vi "Assign Y Coordinate and Width.vi"(5 "Width Padding":i32, 7 "[user-specified font]":T5, 8 "Leaf Width":i32=16, 9 "Row Gap":i32=40, 10 "Max Height per Row":dbl[](array[numeric]), 11 "Tree with Heights in":T1) -> (3 "Decision Tree Out":T1)   [LabVIEW 2025]
uses:
  Types/Decision Tree.ctl
  Types/Sequencing Tree Node.ctl
  Types/Single Cmd Info.ctl
  <vilib>/picture/picture.llb/imagedata.ctl
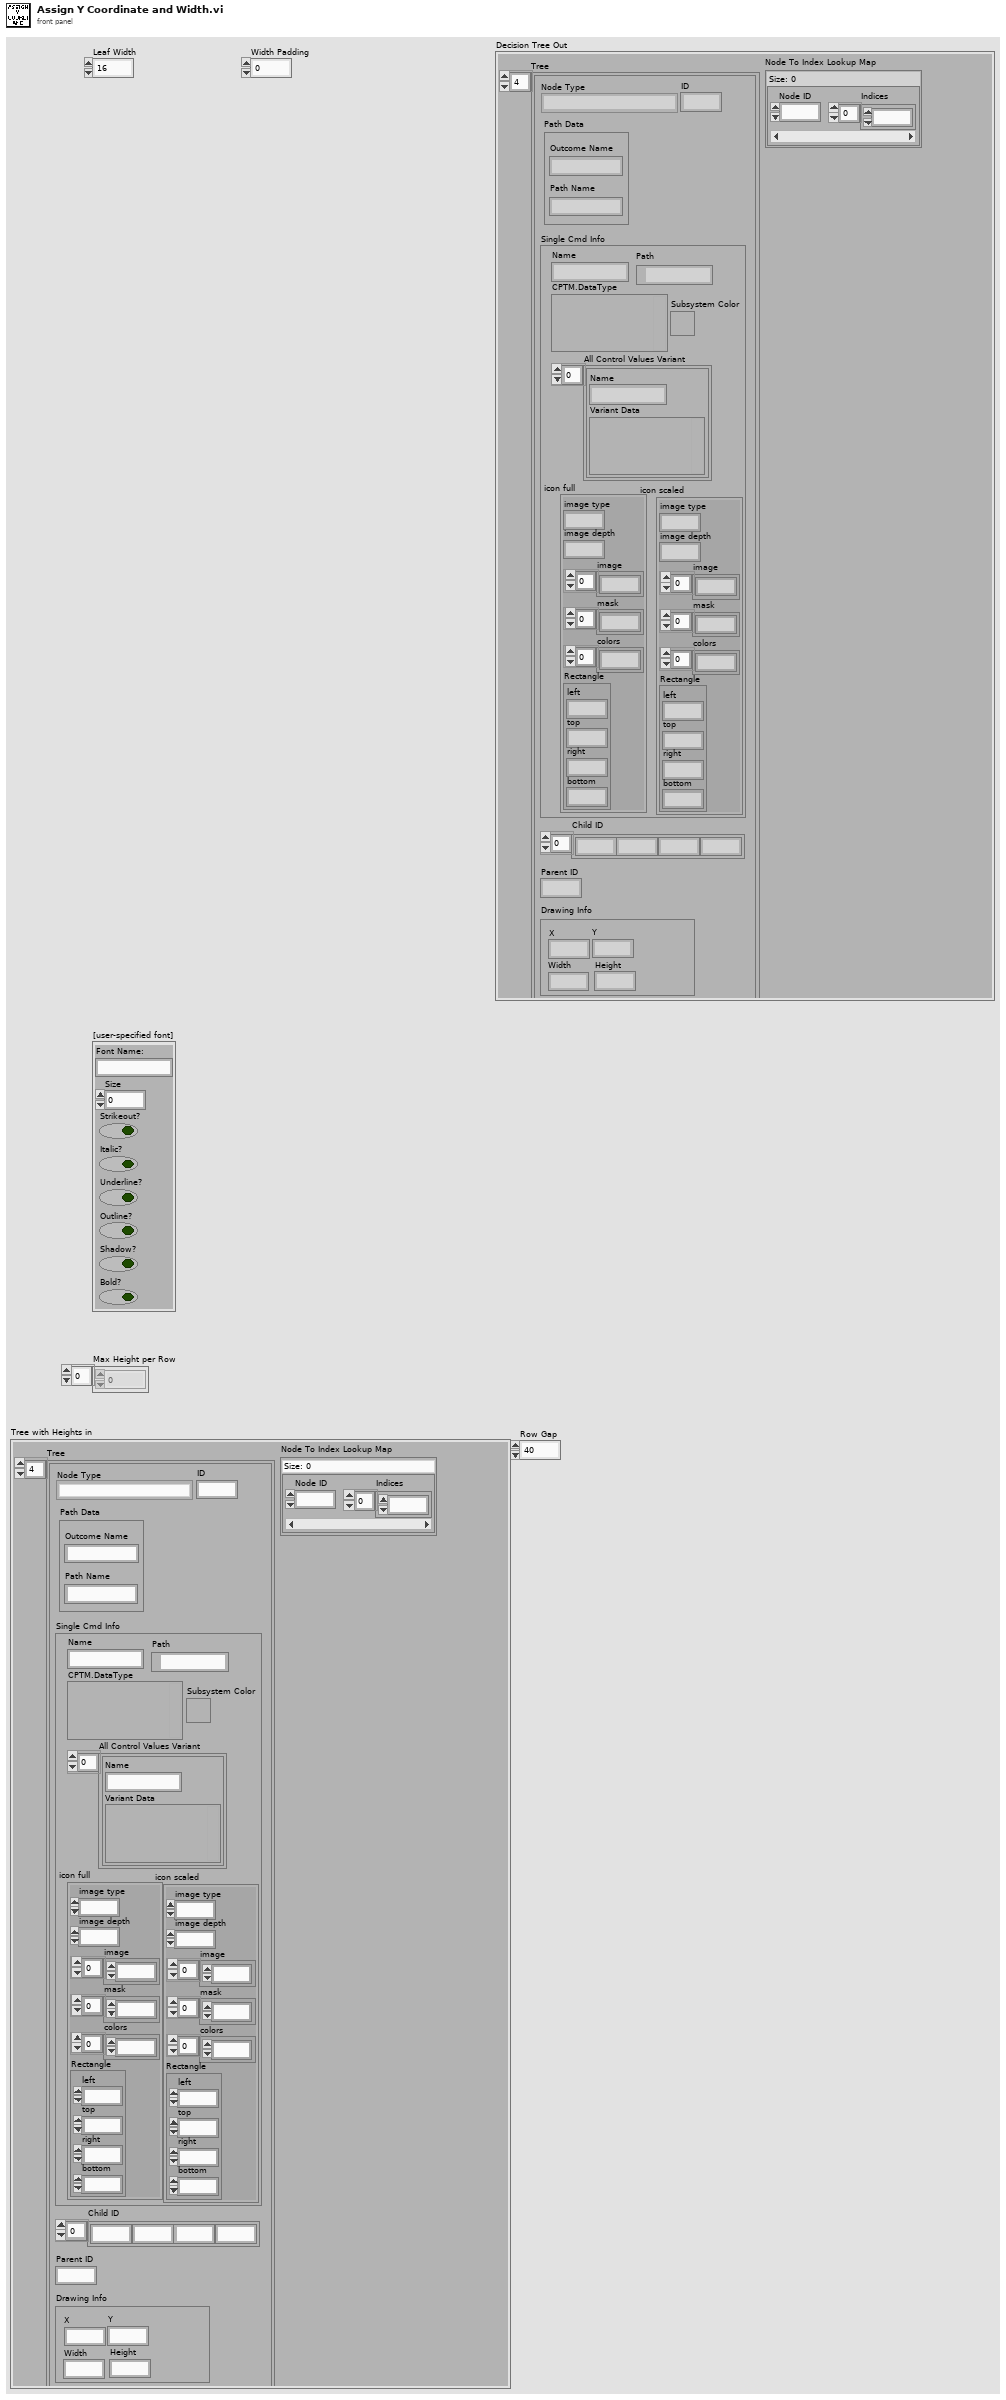
[diagram p1: front panel]
types:
  T1 = typedef "Decision Tree.ctl" = cluster{"Tree":T2[], "Node To Index Lookup Map":map{i16, i16[]}}
  T2 = typedef "Sequencing Tree Node.ctl" = cluster{"Node Type":enum16{"Path", "Command", "Leaf"}, "ID":i16, "Path Data":cluster{"Path Name":string, "Outcome Name":string}, "Single Cmd Info":T3, "Child ID":i32[], "Parent ID":i32, "Drawing Info":cluster{"X":i32, "Y":i32, "Width":i32, "Height":i32}}
  T3 = typedef "Single Cmd Info.ctl" = cluster{"Name":string, "CPTM.DataType":variant, "All Control Values Variant":cluster{"Name":string, "Variant Data":variant}[], "icon full":T4, "icon scaled":T4, "Path":path, "Subsystem Color":u32}
  T4 = typedef "imagedata.ctl" = cluster{"image type":i32, "image depth":i32, "image":u8[], "mask":u8[], "colors":u32[], "Rectangle":cluster{"left":i16, "top":i16, "right":i16, "bottom":i16}}
  T5 = cluster{"Font Name:":string, "Size":i16, "Strikeout?":bool, "Italic?":bool, "Underline?":bool, "Outline?":bool, "Shadow?":bool, "Bold?":bool}
  T6 = enum16{"User-specified Font", "Application Font", "System Font", "Dialog Font"}
  T7 = cluster{"Path Name":string, "Outcome Name":string}
  T8 = cluster{"X":i32, "Y":i32, "Width":i32, "Height":i32}
  T9 = cluster{"left":i16, "top":i16, "right":i16, "bottom":i16}
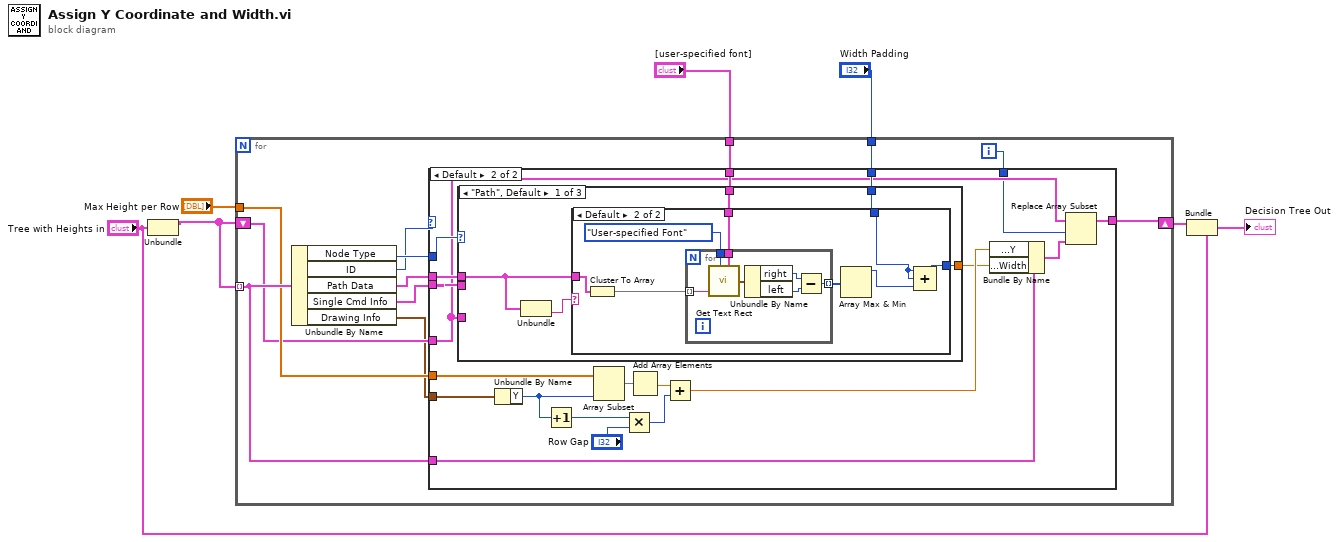
[diagram p0: block diagram]
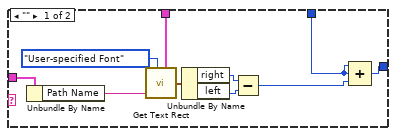
[diagram p3: hidden frame]
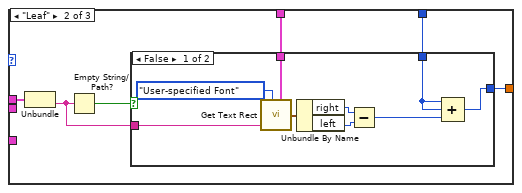
[diagram p4: hidden frame]
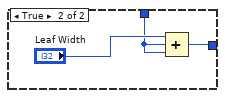
[diagram p5: hidden frame]
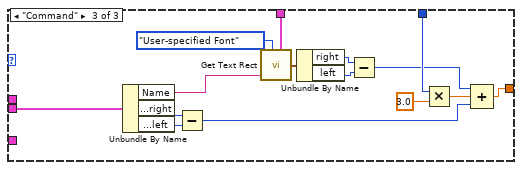
[diagram p6: hidden frame]
diagram:
  n1 = Unbundle("Tree with Heights in") -> ("Tree"=w4:T2[])  [unwired: 1 out]
  n2 = for {
    tunnel: w4 -> [w18] mode=indexing
    tunnel: "Max Height per Row" -> [w17]
    tunnel: "Width Padding" -> [w15]
    tunnel: "[user-specified font]" -> [w14]
    shift-right: [w11] -> w2
    shift-left: w4 -> [w12]
    i -> [w8]
    n3 = Unbundle By Name(w18) -> ("Node Type"=w19:enum16{"Path", "Command", "Leaf"}, "ID"=w10:i16, "Path Data"=w13:T7, "Single Cmd Info"=w16:T3, "Drawing Info"=w9:T8)
    n4 = case shown="Default" w10 {
      tunnel: w19 -> [_ w40]
      tunnel: w18 -> [_ w39]
      tunnel: w9 -> [_ w38]
      tunnel: w17 -> [_ w37]
      tunnel: w16 -> [_ w31]
      tunnel: w15 -> [_ w30]
      tunnel: w14 -> [_ w29]
      tunnel: w13 -> [_ w27]
      tunnel: w12 -> [w20 w26]
      tunnel: [w20 w24] -> w11
      tunnel: w8 -> [_ w21]
      frame -1 {
      }
      frame Default {
        n5 = case shown="\"Path\", Default" w40 {
          tunnel: w31 -> [_ _ w103]
          tunnel: w30 -> [w45 w72 w99]
          tunnel: w29 -> [w44 w73 w98]
          tunnel: [w43 w74 w92] -> w28
          tunnel: w26 -> [_ _ _]
          tunnel: w27 -> [w42 w76 _]
          frame "Path", Default {
            n6 = Unbundle(w42) -> ("Outcome Name"=w41:string)  [unwired: 1 out]
            n7 = case shown="Default" w41 {
              tunnel: w45 -> [w46 w56]
              tunnel: w44 -> [w51 w62]
              tunnel: w42 -> [w50 w61]
              tunnel: [w48 w58] -> w43
              frame "" {
                n8 = Unbundle By Name(w50) -> ("Path Name"=w49:string)
                n9 = call <vilib>:"Get Text Rect.vi"("desired font(Application)"=T6."User-specified Font", "text"=w49, "[user-specified font]"=w51) -> ("rect"=w54:T9)  [unwired: 6 in]
                n10 = Unbundle By Name(w54) -> ("right"=w53:i16, "left"=w52:i16)
                n11 = Subtract(x=w53, y=w52) -> (x-y=w47:i16)
                n12 = Compound Arithmetic op=ADD(w46, w46, w47) -> (w48:i32)
              }
              frame Default {
                n13 = Cluster To Array(cluster=w61) -> (array=w60:string[])
                n14 = for {
                  tunnel: T6."User-specified Font" ("desired font(Application)") -> [w70]
                  tunnel: [w66] -> w59 mode=indexing
                  tunnel: w62 -> [w65]
                  tunnel: w60 -> [w64] mode=indexing
                  n15 = call <vilib>:"Get Text Rect.vi"("desired font(Application)"=w70, "text"=w64, "[user-specified font]"=w65) -> ("rect"=w69:T9)  [unwired: 6 in]
                  n16 = Unbundle By Name(w69) -> ("right"=w68:i16, "left"=w67:i16)
                  n17 = Subtract(x=w68, y=w67) -> (x-y=w66:i16)
                }
                n18 = Array Max & Min(array=w59) -> (max value=w57:i16)  [unwired: 3 out]
                n19 = Compound Arithmetic op=ADD(w56, w56, w57) -> (w58:i32)
              }
            }
          }
          frame "Leaf" {
            n20 = Unbundle(w76) -> ("Outcome Name"=w71:string)  [unwired: 1 out]
            n21 = Empty String/Path?(string/path=w71) -> (empty?=w75:bool)
            n22 = case shown="False" w75 {
              tunnel: [w79 w87] -> w74
              tunnel: w73 -> [w81 _]
              tunnel: w72 -> [w78 w86]
              tunnel: w71 -> [w77 _]
              frame False {
                n23 = call <vilib>:"Get Text Rect.vi"("desired font(Application)"=T6."User-specified Font", "text"=w77, "[user-specified font]"=w81) -> ("rect"=w84:T9)  [unwired: 6 in]
                n24 = Unbundle By Name(w84) -> ("right"=w83:i16, "left"=w82:i16)
                n25 = Subtract(x=w83, y=w82) -> (x-y=w80:i16)
                n26 = Compound Arithmetic op=ADD(w78, w78, w80) -> (w79:i32)
              }
              frame True {
                n27 = Compound Arithmetic op=ADD("Leaf Width", w86, w86) -> (w87:i32)
              }
            }
          }
          frame "Command" {
            n28 = Unbundle By Name(w103) -> ("Name"=w96:string, "icon scaled.Rectangle.right"=w102:i16, "icon scaled.Rectangle.left"=w101:i16)
            n29 = Subtract(x=w102, y=w101) -> (x-y=w91:i16)
            n30 = call <vilib>:"Get Text Rect.vi"("desired font(Application)"=T6."User-specified Font", "text"=w96, "[user-specified font]"=w98) -> ("rect"=w95:T9)  [unwired: 6 in]
            n31 = Unbundle By Name(w95) -> ("right"=w94:i16, "left"=w93:i16)
            n32 = Subtract(x=w94, y=w93) -> (x-y=w89:i16)
            n33 = Multiply(x=w99, y=3.0) -> (x*y=w90:dbl)
            n34 = Compound Arithmetic op=ADD(w89, w90, w91) -> (w92:dbl)
          }
        }
        n35 = Unbundle By Name(w38) -> ("Y"=w22:i32)
        n36 = Increment(x=w22) -> (x+1=w23:i32)
        n37 = Array Subset(array=w37, length=w22) -> (w36:dbl[])  [unwired: 1 in]
        n38 = Multiply(x=w23, y="Row Gap") -> (x*y=w33:i32)
        n39 = Add Array Elements(numeric array=w36) -> (sum=w35:dbl)
        n40 = Add(x=w35, y=w33) -> (x+y=w32:dbl)
        n41 = Bundle By Name(cluster=w39, "Drawing Info.Y"=w32, "Drawing Info.Width"=w28) -> (w25:T2)
        n42 = Replace Array Subset(array=w26, new element=w25, index=w21) -> (w24:T2[])
      }
    }
  }
  n43 = Bundle(cluster="Tree with Heights in", "Tree"=w2) -> (→"Decision Tree Out":T1)  [unwired: 1 in]
